vi "save_dictinoary_json.vi"(7 "unit_dictionary":variant, 8 "error in (no error)":errorcluster, 11 "json_path":path) -> (0 "error out":errorcluster)   [LabVIEW 2015, in "lv-unit-conversion.lvlib"]
uses:
  lv-unit-conversion.lvlib
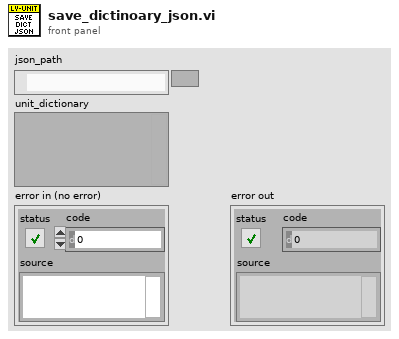
[diagram p1: front panel]
types:
  T1 = typedef "lv-unit-conversion.lvlib/unit.ctl" = cluster{"symbol":string, "name":string, "dimension":string, "is_si_unit":bool, "category":string, "base_unit":string, "conversion_reference":string, "is_exact":bool, "a":dbl, "b":dbl, "c":dbl, "d":dbl, "underlying_def":string, "description":string}
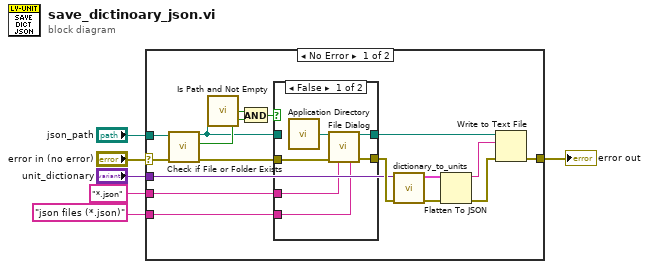
[diagram p0: block diagram]
diagram:
  n1 = case shown="No Error" "error in (no error)" {
    selector: "error in (no error)" -> [w19 w32]
    tunnel: "*.json" ("pattern (all files)") -> [w22 _]
    tunnel: "json files (*.json)" ("pattern label") -> [w21 _]
    tunnel: "json_path" -> [w20 _]
    tunnel: [w7 w32] -> w2
    tunnel: "unit_dictionary" -> [w13 _]
    frame No Error {
      n2 = call <vilib>:"Check if File or Folder Exists.vi"("error in (no error)"=w19, "path"=w20) -> ("error out"=w18:errorcluster, "file or folder exists?"=w17:bool, "dup path"=w14:path)  [unwired: 7 in]
      n3 = call <vilib>:"Is Path and Not Empty.vi"("path"=w14) -> ("Is Path and Not Empty?"=w16:bool)  [unwired: 4 in]
      n4 = And(x=w16, y=w17) -> (x .and. y?=w15:bool)
      n5 = case shown="False" w15 {
        tunnel: w22 -> [w29 _]
        tunnel: w21 -> [w28 _]
        tunnel: [w27 w31] -> w9
        tunnel: [w26 w30] -> w23
        tunnel: w18 -> [w25 w30]
        tunnel: w14 -> [_ w31]
        frame False {
          n6 = call <vilib>:"Application Directory.vi"() -> ("Application Directory"=w24:path)
          n7 = call "File Dialog"("start path"=w24, "error in"=w25, "pattern (all files)"=w29, "pattern label"=w28) -> ("selected path"=w27:path, "error out"=w26:errorcluster)  [unwired: 8 in, 2 out]
        }
        frame True {
        }
      }
      n8 = call "dictionary_to_units.vi"("error in (no error)"=w23, "data_set"=w13) -> ("error out"=w12:errorcluster, "units []"=w11:T1[])  [unwired: 8 in]
      n9 = Flatten To JSON(anything=w11, error in (no error)=w12) -> (JSON string=w8:string, 11:w10:errorcluster)  [unwired: 1 in]
      n10 = Write to Text File(file (use dialog)=w9, text=w8, error in=w10) -> (error out=w7:errorcluster)  [unwired: 1 in, 2 out]
    }
    frame Error {
    }
  }
  "error out" <- w2
